vi "Analyze.vi"(8 "Error In":errorcluster, 10 "LHW-DataCollection":refnum<class "LHW-DataCollection.lvclass">, 11 "LHW-Analysis-Actor in":refnum<class "LHW-Analysis-Actor.lvclass">) -> (0 "Error Out":errorcluster, 3 "LHW-Analysis-Actor out":refnum<class "LHW-Analysis-Actor.lvclass">)   [LabVIEW 2014, in "LHW-Analysis.lvlib" / "LHW-Analysis-Actor.lvclass"]
doc: "Analyze received LHW-DataCollection, append result and update caller."
uses:
  LHW-Analysis-Actor.lvclass
  Classes/LHW-Data/LHW-DataCollection/LHW-DataCollection.lvclass
  <vilib>/ActorFramework/Actor/Actor.lvclass/Actor.ctl
  LHW-GUI-Actor Messages/Update LHW Data Msg/Update LHW Data Msg.lvclass/Update LHW Data Msg.ctl
  <vilib>/ActorFramework/Message Enqueuer/Message Enqueuer.lvclass/Message Enqueuer.ctl
  <vilib>/ActorFramework/Message Enqueuer/Enqueue.vi
  <vilib>/ActorFramework/Message Priority Queue/Priority Enqueue.vi
  <vilib>/ActorFramework/Message Enqueuer/Message Enqueuer.lvclass
  LHW-GUI-Actor Messages/Update LHW Data Msg/Update LHW Data Msg.lvclass
  <vilib>/ActorFramework/Actor/Actor.lvclass
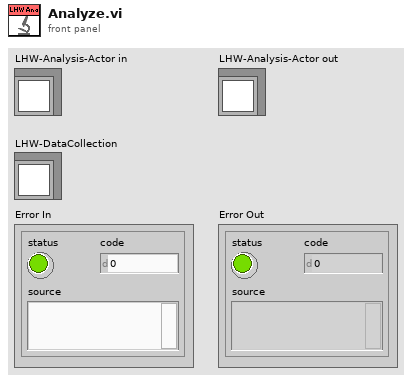
[diagram p1: front panel]
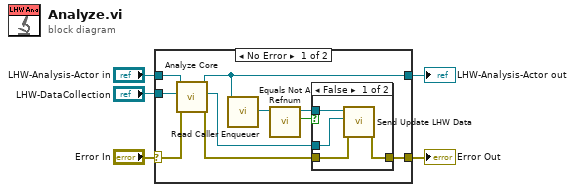
[diagram p0: block diagram]
diagram:
  n1 = case shown="No Error" "Error In" {
    selector: "Error In" -> [w9 w21]
    tunnel: [w12 w21] -> w4
    tunnel: [w10 w20] -> w2
    tunnel: "LHW-Analysis-Actor in" -> [w11 w20]
    tunnel: "LHW-DataCollection" -> [w7 _]
    frame No Error {
      n2 = call-dynamic "Analyze Core.vi"("Error In"=w9, "LHW-DataCollection in"=w7, "LHW-Analysis-Actor in"=w11) -> ("Error Out"=w8:errorcluster, "LHW-DataCollection out"=w6:refnum<class "LHW-DataCollection.lvclass">, "LHW-Analysis-Actor out"=w10:refnum<class "LHW-Analysis-Actor.lvclass">)  [unwired: 6 in]
      n3 = call <vilib>:"Read Caller Enqueuer.vi"("Actor"=w10) -> ("Caller Enqueuer"=w14:refnum<class "Message Enqueuer.lvclass">)  [unwired: 10 in]
      n4 = call <vilib>:"Equals Not A Refnum.vi"("Message Enqueuer"=w14) -> ("Not a refnum?"=w13:bool)  [unwired: 10 in]
      n5 = case shown="False" w13 {
        tunnel: w14 -> [w18 _]
        tunnel: w6 -> [w17 _]
        tunnel: w8 -> [w16 w19]
        tunnel: [w15 w19] -> w12
        frame False {
          n6 = call "Send Update LHW Data.vi"("error in (no error)"=w16, "LHW-DataCollection"=w17, "Message Enqueuer"=w18) -> ("error out"=w15:errorcluster)  [unwired: 7 in, 1 out]
        }
        frame True {
        }
      }
    }
    frame Error {
    }
  }
  "Error Out" <- w4
  "LHW-Analysis-Actor out" <- w2
